vi "PathlossConfig.vi"(8 "error in (no error)":errorcluster, 11 "PathlossConfig":T2={"PathlossFilePath"=path "", "Pathloss Table Name"="", "PhyPort"=enum."Port5"}) -> (0 "error out":errorcluster, 3 "PahtlossCMD":string[](array[string]))   [LabVIEW 2015]
uses:
  PhyPort.ctl
  <vilib>/Utility/file.llb/Read Delimited Spreadsheet (DBL).vi
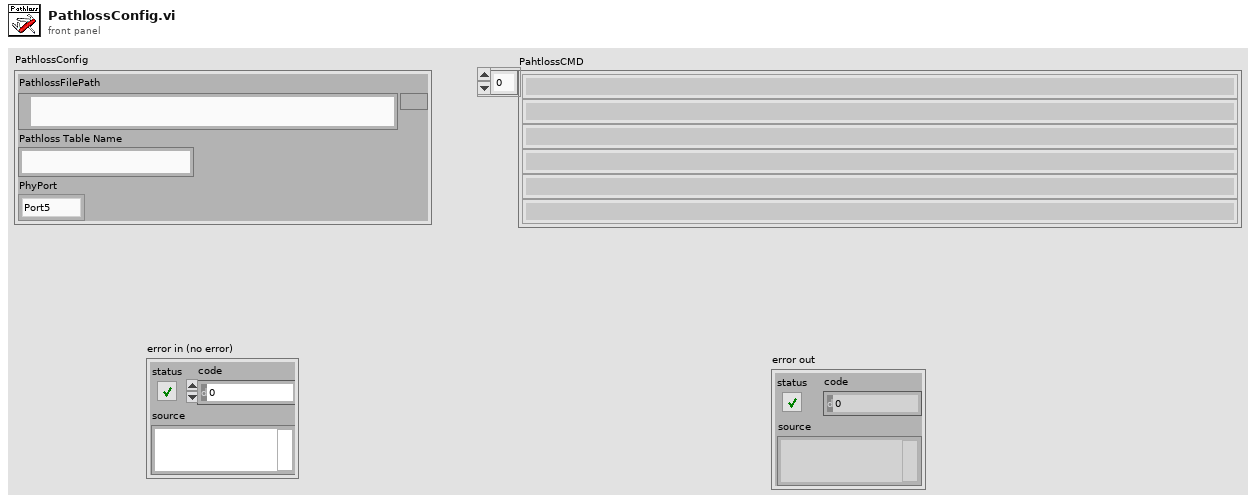
[diagram p1: front panel]
types:
  T1 = typedef "PhyPort.ctl" = enum16{"Port0", "Port1", "Port2", "Port3", "Port4", "Port5", "Port6", "Port7"}
  T2 = cluster{"PathlossFilePath":path, "Pathloss Table Name":string, "PhyPort":T1}
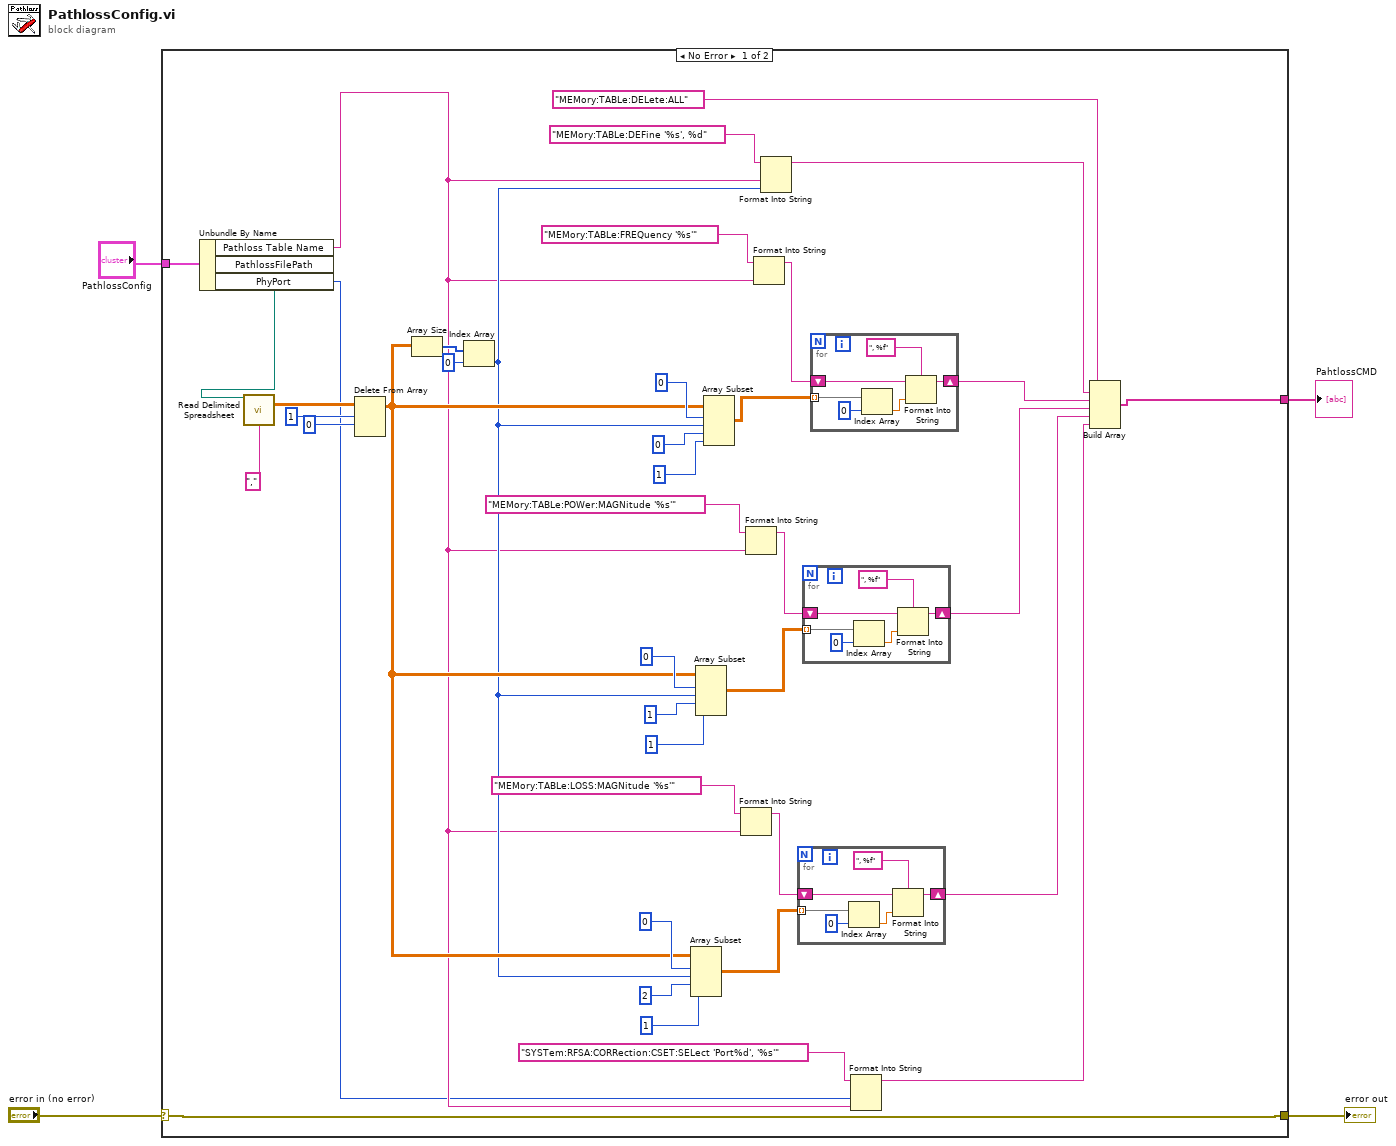
[diagram p0: block diagram]
diagram:
  n1 = case shown="No Error" "error in (no error)" {
    selector: "error in (no error)" -> [w9 w63]
    tunnel: [w9 w63] -> w3
    tunnel: [w10 _] -> w2
    tunnel: "PathlossConfig" -> [w8 _]
    frame No Error {
      n2 = Unbundle By Name(w8) -> ("Pathloss Table Name"=w7:string, "PathlossFilePath"=w6:path, "PhyPort"=w5:T1)
      n3 = call-poly <vilib>:"Read Delimited Spreadsheet.vi"("file path (dialog if empty)"=w6, "delimiter (\\t)"="," ("delimiter (\\t)")) -> ("all rows"=w16:dbl[][])  [unwired: 8 in, 5 out]
      n4 = Delete From Array(array=w16, length=1, index (row)=0) -> (array with subset deleted=w15:dbl[][])  [unwired: 1 in, 1 out]
      n5 = Array Size(array=w15) -> (size(s)=w14:i32[])
      n6 = Index Array(array=w14, index=0) -> (element=w12:i32)
      n7 = Array Subset(array=w15, index (row)=0 ("index"), length (row)=w12, index (col)=2 ("index"), length (col)=1 ("length")) -> (w29:dbl[][])
      n8 = Array Subset(array=w15, index (row)=0 ("index"), length (row)=w12, index (col)=1 ("index"), length (col)=1 ("length")) -> (w36:dbl[][])
      n9 = Array Subset(array=w15, index (row)=0 ("index"), length (row)=w12, index (col)=0 ("index"), length (col)=1 ("length")) -> (w33:dbl[][])
      n10 = Format Into String(format string="MEMory:TABLe:LOSS:MAGNitude '%s'", w7) -> (resulting string=w31:string)  [unwired: 2 in, 1 out]
      n11 = Format Into String(format string="MEMory:TABLe:POWer:MAGNitude '%s'", w7) -> (resulting string=w38:string)  [unwired: 2 in, 1 out]
      n12 = Format Into String(format string="MEMory:TABLe:FREQuency '%s'", w7) -> (resulting string=w34:string)  [unwired: 2 in, 1 out]
      n13 = Format Into String(format string="MEMory:TABLe:DEFine '%s', %d", w7, w12) -> (resulting string=w27:string)  [unwired: 2 in, 1 out]
      n14 = for {
        tunnel: w29 -> [w50] mode=indexing
        shift-right: [w45] -> w24
        shift-left: w31 -> [w48]
        n15 = Index Array(array=w50, index=0) -> (element=w46:dbl)
        n16 = Format Into String(format string=", %f", initial string=w48, w46) -> (resulting string=w45:string)  [unwired: 1 in, 1 out]
      }
      n17 = for {
        tunnel: w36 -> [w62] mode=indexing
        shift-right: [w57] -> w25
        shift-left: w38 -> [w60]
        n18 = Index Array(array=w62, index=0) -> (element=w58:dbl)
        n19 = Format Into String(format string=", %f", initial string=w60, w58) -> (resulting string=w57:string)  [unwired: 1 in, 1 out]
      }
      n20 = for {
        shift-right: [w53] -> w26
        shift-left: w34 -> [w55]
        tunnel: w33 -> [w52] mode=indexing
        n21 = Index Array(array=w52, index=0) -> (element=w51:dbl)
        n22 = Format Into String(format string=", %f", initial string=w55, w51) -> (resulting string=w53:string)  [unwired: 1 in, 1 out]
      }
      n23 = Format Into String(format string="SYSTem:RFSA:CORRection:CSET:SELect 'Port%d', '%s'", w5, w7) -> (resulting string=w19:string)  [unwired: 2 in, 1 out]
      n24 = Build Array("MEMory:TABLe:DELete:ALL", w27, w26, w25, w24, w19) -> (w10:string[])
    }
    frame Error {
    }
  }
  "error out" <- w3
  "PahtlossCMD" <- w2
